vi "Practica4.1_WhileLoop.vi"() -> ()   [LabVIEW 2022 SP3]
panel:
  out "Si se encontró\nNo se encontró":bool
  out "CantidadEjecuciones":dbl
  out "ValorGenerado":dbl
  in  "ValorBuscado":dbl
  # "Anahí Montserrat Vázquez Padilla \nPráctica 04: While loop \n06/02/2024"
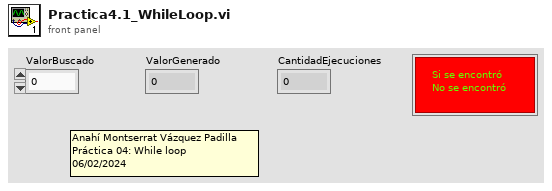
[diagram p1: front panel]
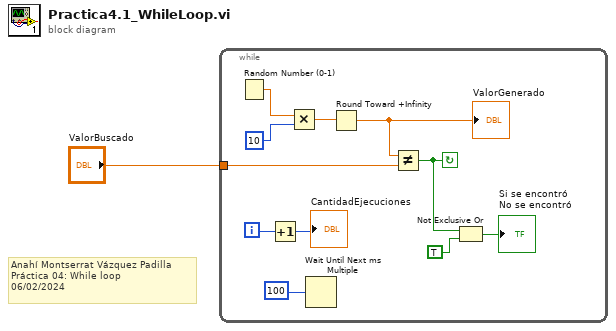
[diagram p0: block diagram]
diagram:
  # "Anahí Montserrat Vázquez Padilla \nPráctica 04: While loop \n06/02/2024"
  n1 = while {
    tunnel: "ValorBuscado" -> [w8]
    i -> [w6]
    stop <- w4 continue-if-true
    n2 = Random Number (0-1)() -> (number: 0 to 1=w11:dbl)
    n3 = Increment(x=w6) -> (x+1=→"CantidadEjecuciones":i32)
    n4 = Multiply(x=w11, y=10) -> (x*y=w10:dbl)
    n5 = Wait Until Next ms Multiple(millisecond multiple=100) -> ()  [unwired: 1 out]
    n6 = Round Toward +Infinity(x=w10) -> (ceil(x): smallest int >= x=w9:dbl)
    "ValorGenerado" <- w9
    n7 = Not Equal?(x=w9, y=w8) -> (x != y?=w4:bool)
    n8 = Not Exclusive Or(1:TRUE, 2:w4) -> (0:→"Si se encontró\nNo se encontró":bool)
  }
